vi "Get Array Size.vi"(8 "error in (no error)":errorcluster, 11 "Array Value":variant) -> (0 "error out":errorcluster, 3 "Array Size":i32)   [LabVIEW 2020, in "MacroAssert.lvlib" / "Numeric Assertion.lvclass"]
doc: "Gets the size of the array contained in the <B>Array Value</B> variant."
uses:
  Numeric Assertion.lvclass
  Numeric Assertion.lvclass/Numeric Assertion.ctl
  SubVIs/Custom Errors/Custom Errors.lvlib
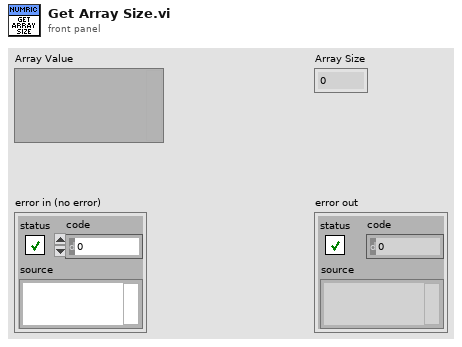
[diagram p1: front panel]
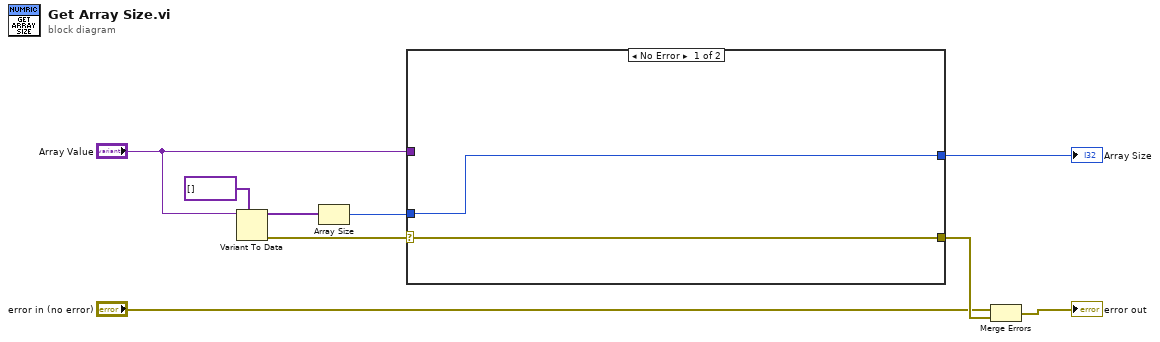
[diagram p0: block diagram]
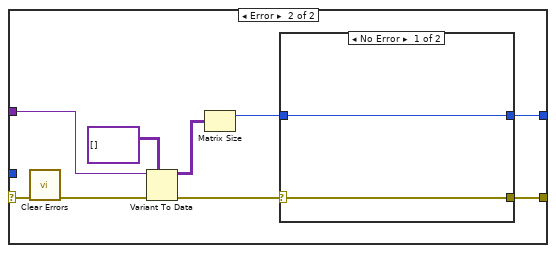
[diagram p2: hidden frame]
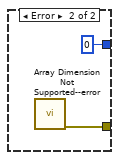
[diagram p3: hidden frame]
diagram:
  n1 = Variant To Data(type=variant[] [], Variant="Array Value") -> (data=w8:variant[], error out=w7:errorcluster)  [unwired: 1 in]
  n2 = Array Size(array=w8) -> (size(s)=w5:i32)
  n3 = case shown="No Error" w7 {
    selector: w7 -> [w10 w19]
    tunnel: "Array Value" -> [_ w18]
    tunnel: [w11 w13] -> w6
    tunnel: w5 -> [w11 _]
    tunnel: [w10 w12] -> w4
    frame No Error {
    }
    frame Error {
      n4 = call <vilib>:"Clear Errors.vi"("error in (no error)"=w19) -> ("error out"=w16:errorcluster)  [unwired: 5 in, 1 out]
      n5 = Variant To Data(error in=w16, type=variant[][] [], Variant=w18) -> (data=w17:variant[][], error out=w15:errorcluster)
      n6 = Matrix Size(0:w17) -> (1:w14:i32)  [unwired: 1 out]
      n7 = case shown="No Error" w15 {
        selector: w15 -> [w21 _]
        tunnel: w14 -> [w22 _]
        tunnel: [w22 0 ("number of columns")] -> w13
        tunnel: [w21 w23] -> w12
        frame No Error {
        }
        frame Error {
          n8 = call "Array Dimension Not Supported--error.vi"() -> ("error out"=w23:errorcluster)  [unwired: 11 in]
        }
      }
    }
  }
  "Array Size" <- w6
  n9 = Merge Errors("error in (no error)", w4) -> (→"error out":errorcluster)
